vi "Frame&Parity Cancel.vi"(8 "error in (no error)":errorcluster={"status"=TRUE, "code"=-1073807339, "source"="VISA Read in Read RPM.vi->LV2017CP.vi"}, 11 "Error Cancellation (Def:On)":bool=TRUE) -> (0 "error out":errorcluster={"status"=TRUE, "code"=-1073807339, "source"="VISA Read in Read RPM.vi->LV2017CP.vi"})   [LabVIEW 2016]
uses:
  <vilib>/Utility/error.llb/DialogType.ctl
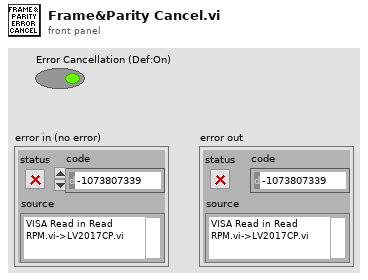
[diagram p1: front panel]
types:
  T1 = typedef "DialogType.ctl" = u16
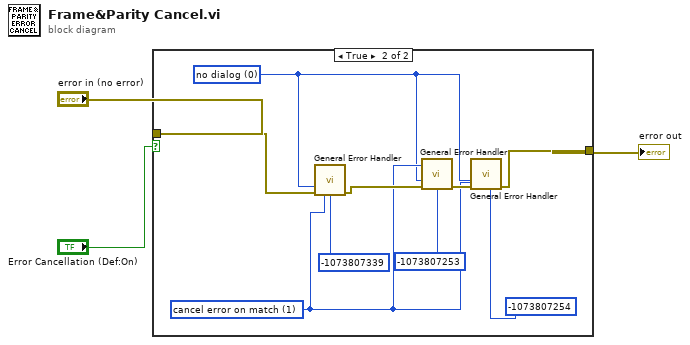
[diagram p0: block diagram]
diagram:
  n1 = case shown="True" "Error Cancellation (Def:On)" {
    tunnel: "error in (no error)" -> [w4 w9]
    tunnel: [w4 w11] -> w1
    frame False {
    }
    frame True {
      w5 = T1 0 items=["no dialog", "OK message", "continue or stop message", "OK message + warnings", "continue/stop + warnings"] ("type of dialog (OK msg:1)")
      w6 = 1 items=["no exception", "cancel error on match", "set error on match"] ("[exception action] (none:0)")
      n2 = call <vilib>:"General Error Handler.vi"("type of dialog (OK msg:1)"=w5, "error in (no error)"=w9, "[exception action] (none:0)"=w6, "[exception code]"=-1073807339) -> ("error out"=w8:errorcluster)  [unwired: 7 in, 4 out]
      n3 = call <vilib>:"General Error Handler.vi"("type of dialog (OK msg:1)"=w5, "error in (no error)"=w8, "[exception action] (none:0)"=w6, "[exception code]"=-1073807253) -> ("error out"=w12:errorcluster)  [unwired: 7 in, 4 out]
      n4 = call <vilib>:"General Error Handler.vi"("type of dialog (OK msg:1)"=w5, "error in (no error)"=w12, "[exception action] (none:0)"=w6, "[exception code]"=-1073807254 ("[exception code] 2")) -> ("error out"=w11:errorcluster)  [unwired: 7 in, 4 out]
    }
  }
  "error out" <- w1
